vi "downramp.vi"(11 "number of steps":i32=50) -> (3 "downramp array":dbl[](array[numeric]))   [LabVIEW 2020]
uses:
  File Exists - Scalar__ogtk.vi
  Read Delimited Spreadsheet (DBL).vi
  Write Delimited Spreadsheet (DBL).vi
panel:
  out "downramp array 3":dbl[](graph)
  out "downramp array 2":dbl[](graph)
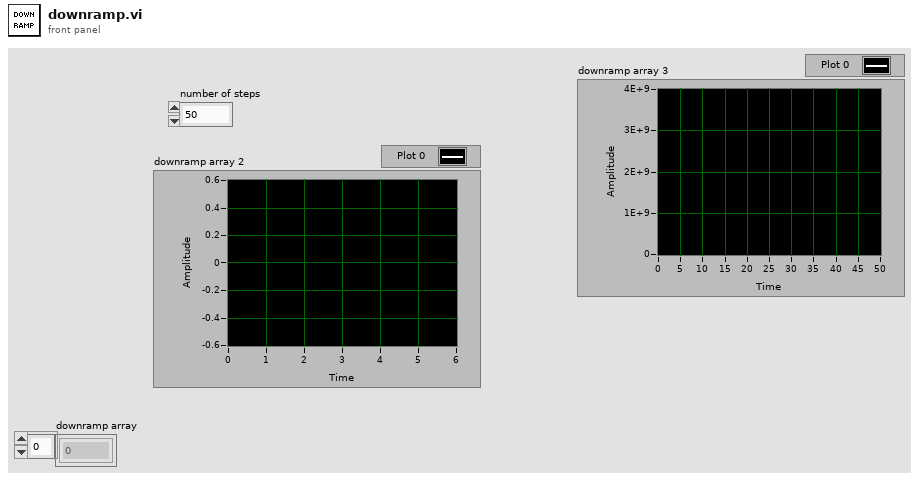
[diagram p1: front panel]
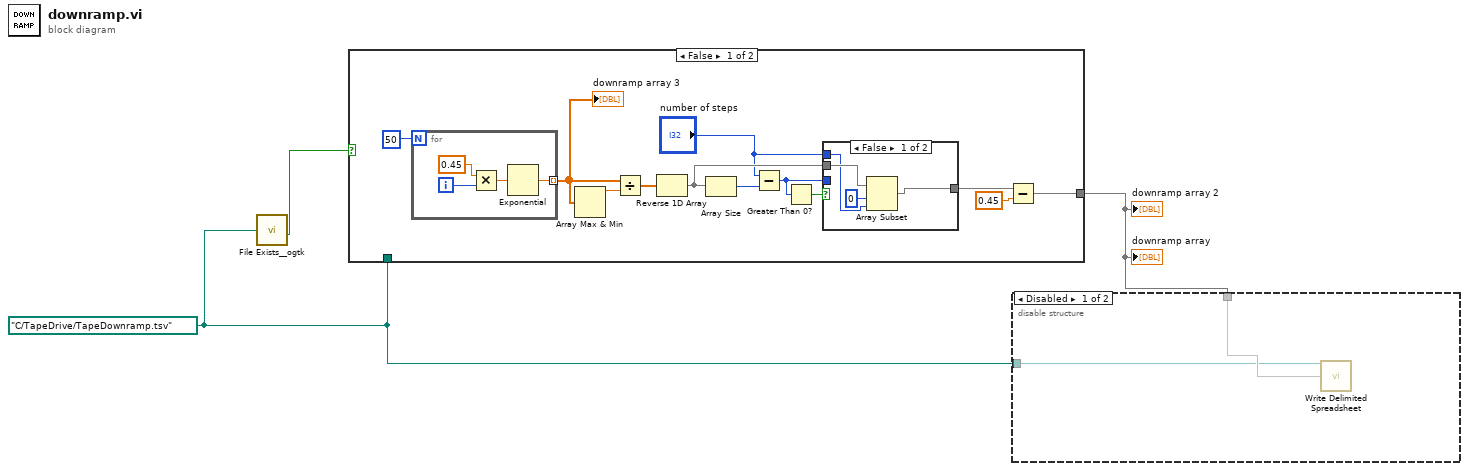
[diagram p0: block diagram]
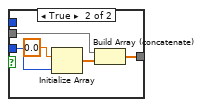
[diagram p2: hidden frame]
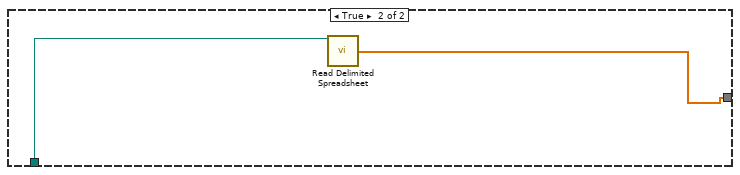
[diagram p3: hidden frame]
diagram:
  w2 = path "C:/TapeDrive/TapeDownramp.tsv" ("file path (dialog if empty)")
  n1 = call-poly "File Exists__ogtk.vi"("file path"=w2) -> ("exists"=w1:bool)  [unwired: 6 in, 1 out]
  n2 = case shown="False" w1 {
    tunnel: [w4 w29] -> w3
    tunnel: w2 -> [_ w30]
    frame False {
      n3 = for {
        N: 50 -> [_]
        tunnel: [w28] -> w13 mode=indexing
        i -> [w27]
        n4 = Multiply(x=0.45, y=w27) -> (x*y=w25:dbl)
        n5 = Exponential(1:w25) -> (0:w28:dbl)
      }
      "downramp array 3" <- w13
      n6 = Array Max & Min(array=w13) -> (max value=w15:dbl)  [unwired: 3 out]
      n7 = Divide(x=w13, y=w15) -> (x/y=w12:dbl[])
      n8 = Reverse 1D Array(array=w12) -> (reversed array=w10:dbl[])
      n9 = Array Size(array=w10) -> (size(s)=w8:i32)
      n10 = Subtract(x="number of steps", y=w8) -> (x-y=w7:i32)
      n11 = Greater Than 0?(x=w7) -> (x > 0?=w6:bool)
      n12 = case shown="False" w6 {
        tunnel: w10 -> [w19 w24]
        tunnel: [w17 w23] -> w9
        tunnel: w7 -> [_ w22]
        tunnel: "number of steps" -> [w16 _]
        frame False {
          n13 = Array Subset(array=w19, index=0, length=w16) -> (w17:dbl[])
        }
        frame True {
          n14 = Initialize Array(0.0 ("element"), w22) -> (w20:dbl[])
          n15 = Build Array (concatenate)(w24, w20) -> (w23:dbl[])
        }
      }
      n16 = Subtract(x=w9, y=0.45 ("x")) -> (x-y=w4:dbl[])
    }
    frame True {
      n17 = call-poly "Read Delimited Spreadsheet.vi"("file path (dialog if empty)"=w30) -> ("first row"=w29:dbl[])  [unwired: 9 in, 5 out]
    }
  }
  "downramp array" <- w3
  "downramp array 2" <- w3
  n18 = disable-structure shown="Disabled" {
    disable-tunnel: w3 -> [w32 _]
    disable-tunnel: w2 -> [w31 _]
    frame Disabled {
      n19 = call-poly "Write Delimited Spreadsheet.vi"("file path (dialog if empty)"=w31, "1D data"=w32) -> ()  [unwired: 12 in, 2 out]
    }
    frame Enabled {
    }
  }
